vi "client.echo.vi"(8 "error in (no error)":errorcluster, 10 "value in":string, 11 "TCP Network Connection in":refnum<k5>) -> (0 "error out":errorcluster, 2 "value out":string, 3 "TCP Network Connection out":refnum<k5>)   [LabVIEW 2017]
uses:
  <vilib>/NI/JSON Support for LabVIEW/JSON Value/New JSON Value/New JSON (String).vi
  <vilib>/NI/NI JSONRPC Server Framework/Classes/Client/Format Client Request (Auto-Increment).vi
  <vilib>/NI/JSON Support for LabVIEW/JSON Value/Read Value/Read value (String).vi
  <vilib>/NI/NI JSONRPC Server Framework/Classes/Client/JSONRPC Client.lvclass
  <vilib>/NI/JSON Support for LabVIEW/JSON Value/JSON Value.lvclass
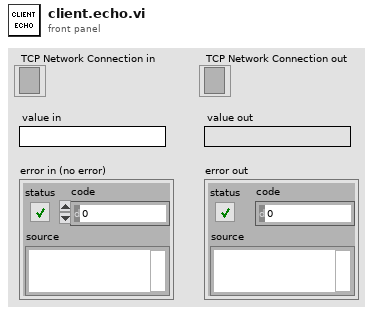
[diagram p1: front panel]
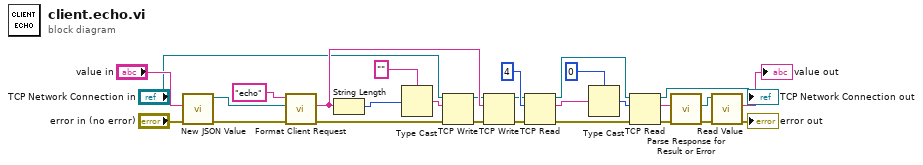
[diagram p0: block diagram]
diagram:
  n1 = call-poly <vilib>:"New JSON Value.vi"("error in (no error)"="error in (no error)", "value"="value in") -> ("error out"=w18:errorcluster, "JSON Value out"=w3:refnum<class "JSON Value.lvclass">)  [unwired: 8 in]
  n2 = call-poly <vilib>:"Format Client Request.vi"("error in (no error)"=w18, "JSON Value in"=w3, "method"="echo") -> ("error out"=w17:errorcluster, "Request String"=w23:string)  [unwired: 7 in]
  n3 = String Length(string=w23) -> (length=w4:i32)
  n4 = Type Cast(type="", x=w4) -> (*(type *) &x=w5:string)
  n5 = TCP Write(connection ID="TCP Network Connection in", data in=w5, error in (no error)=w17) -> (connection ID out=w7:refnum<k5>, error out=w16:errorcluster)  [unwired: 1 in, 1 out]
  n6 = TCP Write(connection ID=w7, data in=w23, error in (no error)=w16) -> (connection ID out=w8:refnum<k5>, error out=w15:errorcluster)  [unwired: 1 in, 1 out]
  n7 = TCP Read(connection ID=w8, bytes to read=4, error in (no error)=w15) -> (connection ID out=w13:refnum<k5>, data out=w11:string, error out=w14:errorcluster)  [unwired: 2 in]
  n8 = Type Cast(type=0 ("length"), x=w11) -> (*(type *) &x=w12:i32)
  n9 = TCP Read(connection ID=w13, bytes to read=w12, error in (no error)=w14) -> (connection ID out=→"TCP Network Connection out":refnum<k5>, data out=w21:string, error out=w20:errorcluster)  [unwired: 2 in]
  n10 = call <vilib>:"Parse Response for Result or Error.vi"("error in"=w20, "Response String In"=w21) -> ("error out"=w27:errorcluster, "JSON Value out"=w25:refnum<class "JSON Value.lvclass">)  [unwired: 7 in, 1 out]
  n11 = call-poly <vilib>:"Read Value.vi"("error in (no error)"=w27, "JSON String in"=w25) -> ("error out"=→"error out":errorcluster, "value"=→"value out":string)  [unwired: 7 in, 1 out]
